vi "PM9_TCP_DEG-UNITS.vi"(0 "VISA":refnum<visa-resource-name>="TCPIP0::169.254.70.190::502::SOCKET", 5 "connection ID":refnum<k5>, 11 "error in (no error)":errorcluster, 12 "Units[C|F]":i32(ring) items=["°C", "°F"], 13 "Close TCP(t)":bool, 14 "RO|WO":i32(ring) items=["RO", "WO"]) -> (3 "output":string, 4 "visa out":refnum<visa-resource-name>, 6 "connection ID out":refnum<k5>, 15 "error out":errorcluster)   [LabVIEW 2018]
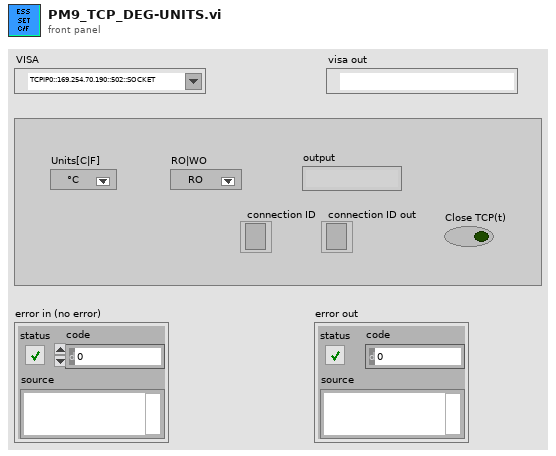
[diagram p1: front panel]
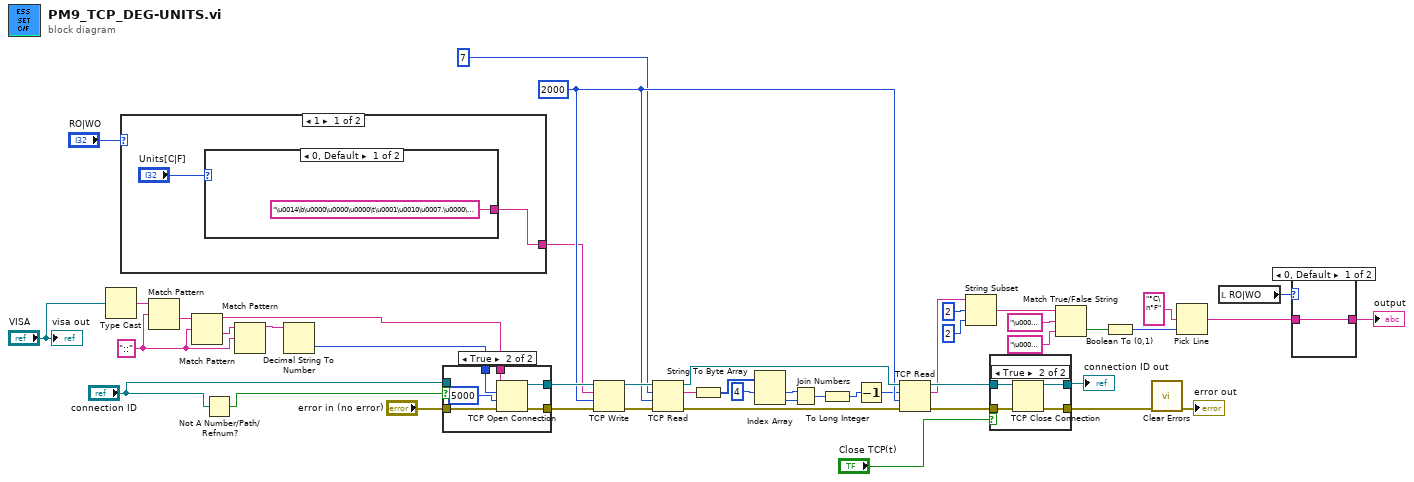
[diagram p0: block diagram]
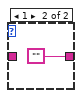
[diagram p4: hidden frame]
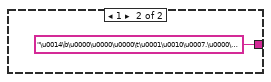
[diagram p5: hidden frame]
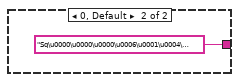
[diagram p6: hidden frame]
diagram:
  w18 = "::" ("search string/char (-)")
  w38 = 2000 ("timeout ms (25000)")
  n1 = Type Cast(x="VISA") -> (*(type *) &x=w21:string)  [unwired: 1 in]
  n2 = case shown="1" "RO|WO" {
    tunnel: [w49 "Sq\u0000\u0000\u0000\u0006\u0001\u0004\u0007.\u0000\u0002" ("data in")] -> w28
    frame 1 {
      n3 = case shown="0, Default" "Units[C|F]" {
        tunnel: ["\u0014\b\u0000\u0000\u0000\t\u0001\u0010\u0007.\u0000\u0001\u0002\u0000\u000f" ("data in") "\u0014\b\u0000\u0000\u0000\t\u0001\u0010\u0007.\u0000\u0001\u0002\u0000\u001e" ("data in")] -> w49
        frame 0, Default {
        }
        frame 1 {
        }
      }
    }
    frame 0, Default {
    }
  }
  n4 = Match Pattern(string=w21, regular expression=w18) -> (after substring=w20:string)  [unwired: 1 in, 3 out]
  n5 = Match Pattern(string=w20, regular expression=w18) -> (before substring=w15:string, after substring=w19:string)  [unwired: 1 in, 2 out]
  n6 = Not A Number/Path/Refnum?(number/path/refnum="connection ID") -> (NaN/Path/Refnum?=w3:bool)
  n7 = Match Pattern(string=w19, regular expression=w18) -> (before substring=w17:string)  [unwired: 1 in, 3 out]
  n8 = Decimal String To Number(string=w17) -> (number=w16:i32)  [unwired: 2 in, 1 out]
  n9 = case shown="True" w3 {
    tunnel: [w54 w60] -> w47
    tunnel: [w53 w59] -> w46
    tunnel: w16 -> [_ w58]
    tunnel: w15 -> [_ w57]
    tunnel: "error in (no error)" -> [w53 w55]
    tunnel: "connection ID" -> [w54 _]
    frame False {
    }
    frame True {
      n10 = TCP Open Connection(address=w57, remote port or service name=w58, timeout ms (60000)=5000, error in (no error)=w55) -> (connection ID=w60:refnum<k5>, error out=w59:errorcluster)  [unwired: 1 in]
    }
  }
  n11 = TCP Write(connection ID=w47, data in=w28, error in (no error)=w46, 9:w38) -> (connection ID out=w42:refnum<k5>, error out=w40:errorcluster)  [unwired: 1 out]
  n12 = TCP Read(connection ID=w42, bytes to read=7, error in (no error)=w40, 9:w38) -> (connection ID out=w41:refnum<k5>, data out=w31:string, error out=w39:errorcluster)  [unwired: 1 in]
  n13 = String To Byte Array(string=w31) -> (unsigned byte array=w32:u8[])
  n14 = Index Array(array=w32, index #1=4 ("index")) -> (element #1=w33:u8, element #2=w34:u8)  [unwired: 1 in]
  n15 = Join Numbers(hi=w33, lo=w34) -> ((hi.lo)=w36:u16)
  n16 = To Long Integer(number=w36) -> (32bit integer=w35:i32)
  n17 = Decrement(x=w35) -> (x-1=w30:i32)
  n18 = TCP Read(connection ID=w41, bytes to read=w30, error in (no error)=w39, 9:w38) -> (connection ID out=w45:refnum<k5>, data out=w29:string, error out=w44:errorcluster)  [unwired: 1 in]
  n19 = String Subset(string=w29, offset (0)=u16 2 ("bytes to read"), length (rest)=u16 2 ("bytes to read")) -> (substring=w14:string)
  n20 = case shown="True" "Close TCP(t)" {
    tunnel: w45 -> [w62 w66]
    tunnel: w44 -> [w61 w65]
    tunnel: [w61 w64] -> w43
    tunnel: [w62 w63] -> w2
    frame False {
    }
    frame True {
      n21 = TCP Close Connection(connection ID=w66, error in (no error)=w65) -> (connection ID out=w63:refnum<k5>, error out=w64:errorcluster)  [unwired: 1 in]
    }
  }
  "connection ID out" <- w2
  n22 = Match True/False String(2:"\u0000\u000f" ("true string"), 3:"\u0000\u001e" ("true string"), 4:w14) -> (0:w11:bool)  [unwired: 1 out]
  n23 = Boolean To (0,1)(Boolean=w11) -> (0, 1=w9:i16)
  n24 = call <vilib>:"Clear Errors.vi"("error in (no error)"=w43) -> ("error out"=→"error out":errorcluster)  [unwired: 5 in, 1 out]
  n25 = Pick Line(multi-line string="°C\n°F", line index=w9) -> (output string=w8:string)  [unwired: 1 in]
  n26 = local read "RO|WO"() -> (w6:i32)
  n27 = case shown="0, Default" w6 {
    tunnel: w8 -> [w67 _]
    tunnel: [w67 ""] -> w7
    frame 0, Default {
    }
    frame 1 {
    }
  }
  "output" <- w7
  "visa out" <- "VISA"
